vi "GenFilenames.vi"(2 "Controller name":string="Unnamed", 3 "Default dir":path=path "T:/PROJECTS/02-ACTIVE/116758_Trapped_Ion_Optical_Frequency_Standards/Technical/Yb+/Science/Temperature control/Data") -> (1 "Log file":path)   [LabVIEW 2015]
doc: "Generate filenames for the data log files"
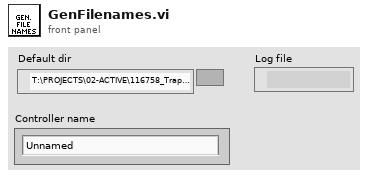
[diagram p1: front panel]
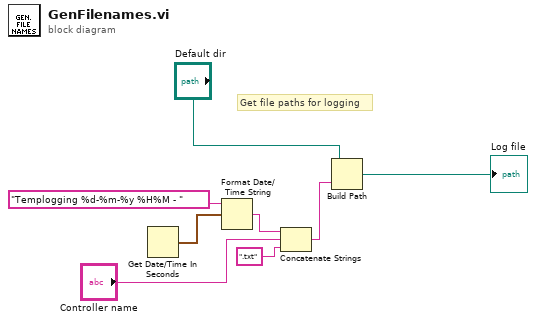
[diagram p0: block diagram]
diagram:
  # "Get file paths for logging"
  n1 = Get Date/Time In Seconds() -> (seconds since 1Jan1904=w3:timestamp)
  n2 = Format Date/Time String(time format string (%c)="Templogging %d-%m-%y %H%M - ", seconds (now)=w3) -> (date/time string=w8:string)  [unwired: 1 in]
  n3 = Concatenate Strings(w8, "Controller name", ".txt") -> (w6:string)
  n4 = Build Path(base path="Default dir", name or relative path=w6) -> (appended path=→"Log file":path)
